vi "Device_Detection.vi"(8 "error in (no error)":errorcluster, 11 "Path":path) -> (0 "error out":errorcluster, 2 "retuen":i32, 3 "Path output":path)   [LabVIEW 2014]
uses:
  Typedef/Hardware Type.ctl
panel:
  out "array":string[](array[string])
  out "array":T1[](array[typedef]) items=["BUS_UNKNOWN_TYPE", "TS_TCP_DEVICE", "XL_USB_DEVICE", "TS_USB_DEVICE", "PEAK_USB_DEVICE", "KVASER_USB_DEVICE", "ZLG_USB_DEVICE", "ICS_USB_DEVICE", "TS_TC1005_DEVICE", "CANABLE_USB_DEVICE", "TS_WIRELESS_OBD", "TS_USB_DEVICE_EX", "IXXAT_USB_DEVICE", "TS_ETH_IF_DEVICE", "TS_USB_IF_DEVICE", "BUS_DEV_TYPE_COUNT"]
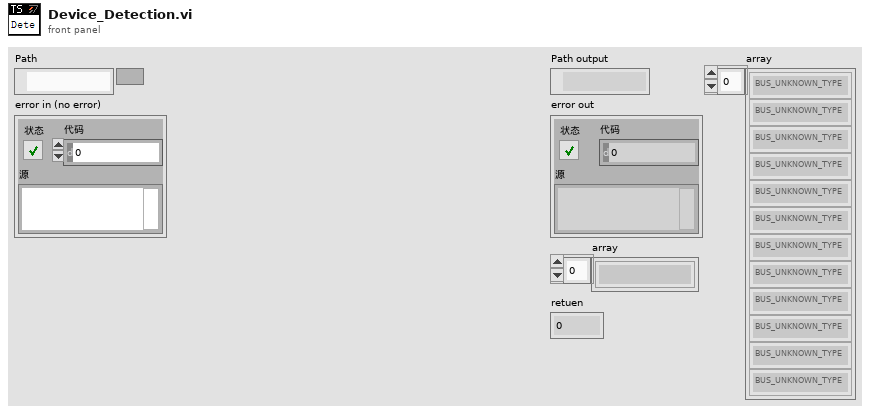
[diagram p1: front panel]
types:
  T1 = typedef "Hardware Type.ctl" = i32
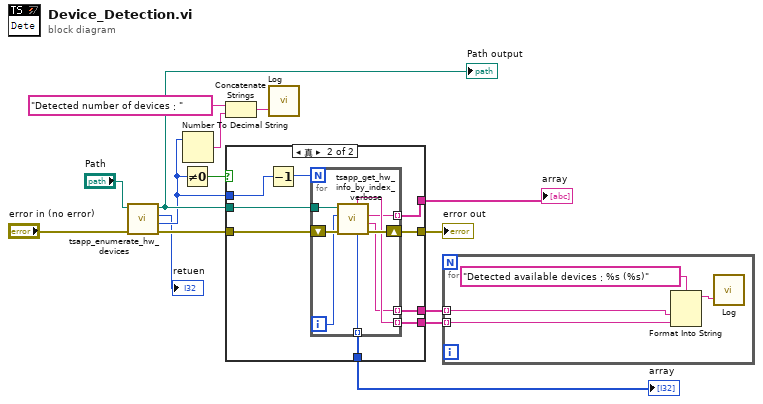
[diagram p0: block diagram]
diagram:
  n1 = call "tsapp_enumerate_hw_devices.vi"("error in (no error)"="error in (no error)", "Path"="Path") -> ("error out"=w12:errorcluster, "ACount"=w2:i32, "retuen"=→"retuen":i32, "Path output"=w7:path)  [unwired: 6 in]
  "Path output" <- w7
  n2 = Not Equal To 0?(x=w2) -> (x != 0?=w11:bool)
  n3 = Number To Decimal String(number=w2) -> (decimal integer string=w13:string)  [unwired: 1 in]
  n4 = Concatenate Strings("Detected number of devices：", w13) -> (w14:string)
  n5 = case shown="真" w11 {
    tunnel: w12 -> [w16 w24]
    tunnel: [w16 w23] -> w5
    tunnel: [_ w22] -> w10
    tunnel: [_ w21] -> w9
    tunnel: w2 -> [_ w20]
    tunnel: w7 -> [_ w19]
    tunnel: [_ w18] -> w3
    tunnel: [_ w17] -> w4
    frame False {
    }
    frame True {
      n6 = Decrement(x=w20) -> (x-1=w25:i32)
      n7 = for {
        N: w25 -> [_]
        shift-right: [w32] -> w23
        shift-left: w24 -> [w33]
        tunnel: [w31] -> w22 mode=indexing
        tunnel: [w30] -> w21 mode=indexing
        tunnel: w19 -> [w29]
        tunnel: [w27] -> w18 mode=indexing
        tunnel: [w26] -> w17 mode=indexing
        i -> [w28]
        n8 = call "tsapp_get_hw_info_by_index_verbose.vi"("error in"=w33, "AIndex"=w28, "路径输入"=w29) -> ("error out"=w32:errorcluster, "DeviceName"=w30:string, "VendorName"=w27:string, "Hardware Type"=w26:T1, "SerialNum"=w31:string)  [unwired: 3 in, 1 out]
      }
    }
  }
  "error out" <- w5
  "array" <- w4
  "array" <- w3
  n9 = call "Log.vi"("Data"=w14) -> ()  [unwired: 3 in]
  n10 = for {
    tunnel: w10 -> [w35] mode=indexing
    tunnel: w9 -> [w36] mode=indexing
    n11 = Format Into String(format string="Detected available devices：%s (%s)", w36, w35) -> (resulting string=w34:string)  [unwired: 2 in, 1 out]
    n12 = call "Log.vi"("Data"=w34) -> ()  [unwired: 3 in]
  }
